vi "Landscape Global.vi"() -> ()   [LabVIEW 2015, in "Defenders.lvclass"]
uses:
  Defenders.lvclass
  Terrain.ctl
  Type Defs/Direction Enum.ctl
  Type Defs/SB Type Defs.lvlib
panel:
  in  "LandScape":cluster{"Terrain":T1, "Direction":T2}[][](array[cluster])
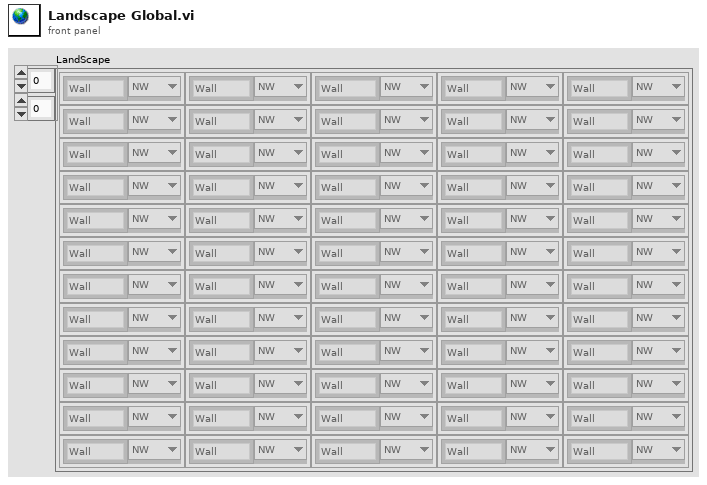
[diagram p1: front panel]
types:
  T1 = typedef "Defenders.lvclass/Terrain.ctl" = enum16{"Wall", "EnemySighted", "EnemyWall", "Mother", "Move", "StagingArea"}
  T2 = typedef "SB Type Defs.lvlib/Direction Enum.ctl" = enum16{"NW", "N", "NE", "E", "SE", "S", "SW", "W"}
diagram:
